vi "Reset.vi"(8 "error in (no error)":errorcluster, 11 "VGC in":refnum<class "PL Inficon VGC.lvclass">) -> (0 "error out":errorcluster, 2 "errors":u16[](array[ring]) items=["no error", "watchdog responded", "task fail error", "FLASH error", "RAM error", "EEPROM error", "display error", "A/D converter error", "UART error", "gauge 1 general error", "gauge 1 id error", "gauge 2 general error", "gauge 2 id error", "gauge 3 general error", "gauge 3 id error"], 3 "VGC out":refnum<class "PL Inficon VGC.lvclass">)   [LabVIEW 2015, in "PL Inficon VGC.lvclass"]
doc: "Resets and returns all present errors."
uses:
  PL Inficon VGC.lvclass
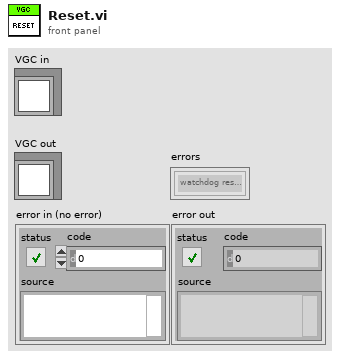
[diagram p1: front panel]
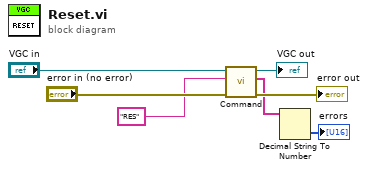
[diagram p0: block diagram]
diagram:
  n1 = call "Command.vi"("error in (no error)"="error in (no error)", "command"="RES", "VGC in"="VGC in") -> ("error out"=→"error out":errorcluster, "response data"=w1:string[], "VGC out"=→"VGC out":refnum<class "PL Inficon VGC.lvclass">)  [unwired: 6 in]
  n2 = Decimal String To Number(string=w1) -> (number=→"errors":i32[])  [unwired: 2 in, 1 out]
